vi "Process.vi"(8 "error in (no error)":errorcluster, 10 "pound in":refnum<class "Pound.lvclass">, 11 "qbus in":refnum<class "Qbus.lvclass">) -> (0 "error out":errorcluster)   [LabVIEW 2015, in "MainController.lvlib"]
doc: "Implements timer tasks that other processes register by sending Qbus messages to those processes."
uses:
  MainController.lvlib
  <vilib>/addons/Qbus/Qbus.lvclass
  <vilib>/NI/Software Watchdog/Pound/Pound.lvclass
  controls/ProcessState.ctl
  <vilib>/drjdpowell/SQLite Library/SQL Connection/Connection.lvclass
  <vilib>/NI/Software Watchdog/Watchdog/Watchdog.lvclass
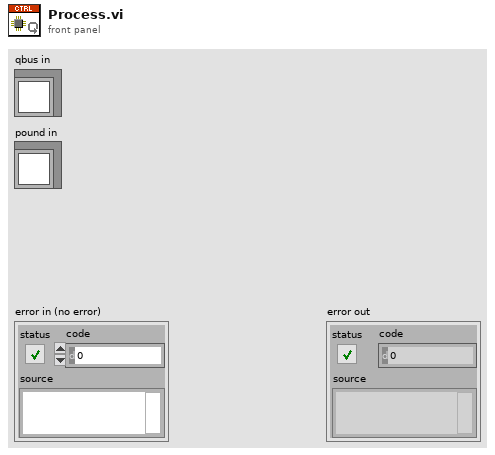
[diagram p1: front panel]
types:
  T1 = typedef "MainController.lvlib/ProcessState.ctl" = cluster{"SQLite Connection":refnum<class "Connection.lvclass">}
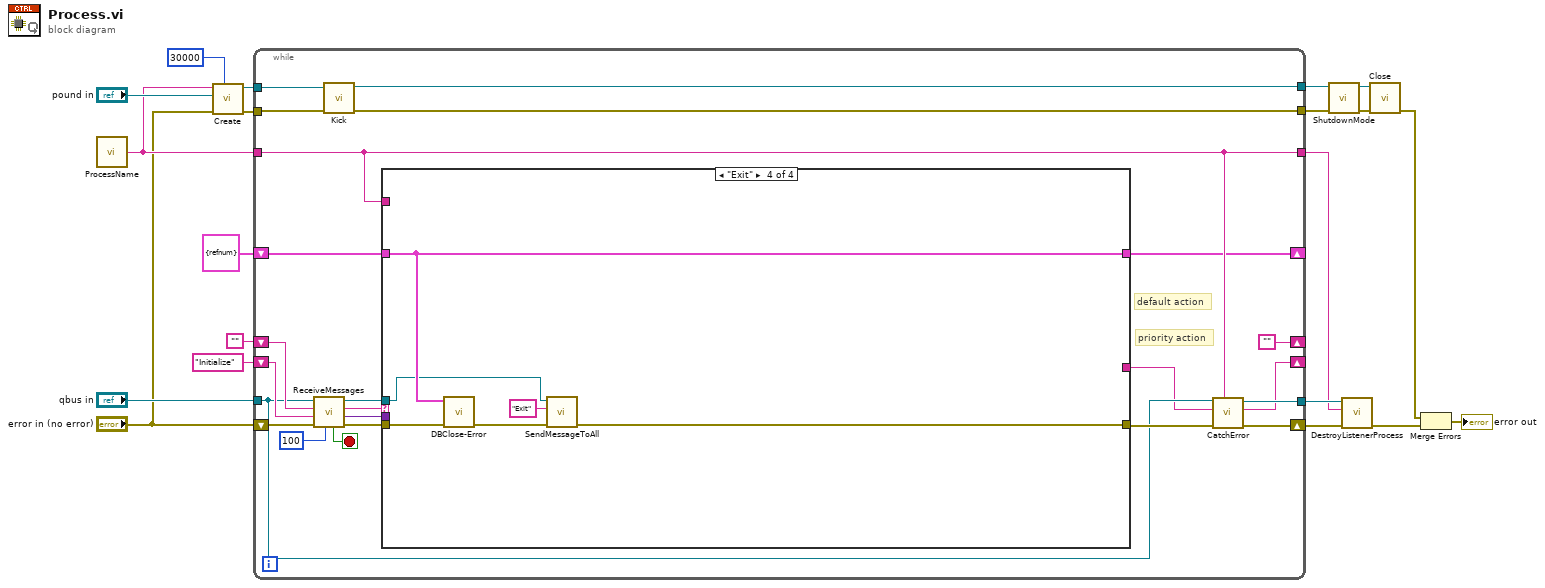
[diagram p0: block diagram]
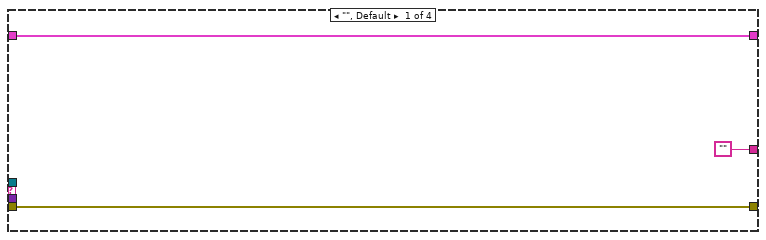
[diagram p2: hidden frame]
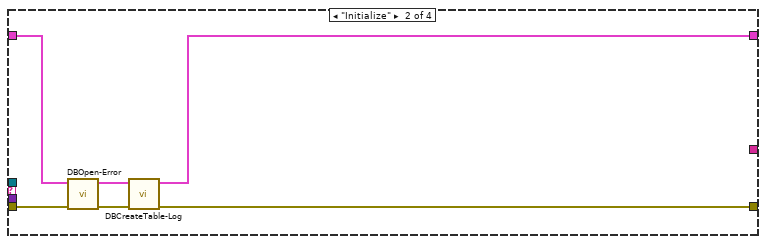
[diagram p3: hidden frame]
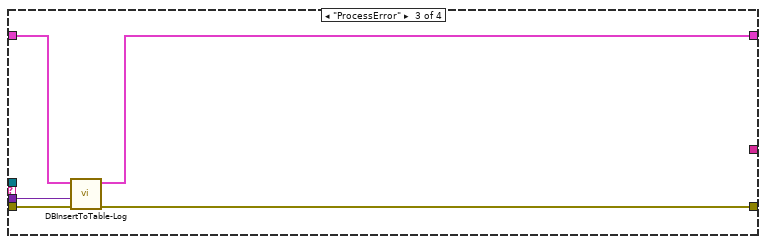
[diagram p4: hidden frame]
diagram:
  n1 = call "ProcessName.vi"() -> ("process name"=w11:string)  [unwired: 5 in]
  n2 = call <vilib>:"Create.vi"("Execution Timeout (ms)"=u32 30000, "error in (no error)"="error in (no error)", "Pound"="pound in", "Name"=w11) -> ("error out"=w13:errorcluster, "Watchdog"=w12:refnum<data-value>)  [unwired: 6 in]
  n3 = while {
    shift-right: [""] -> _
    shift-left: "" -> [w41]
    tunnel: "qbus in" -> [w25]
    tunnel: w11 -> [w32]
    tunnel: [w34] -> w18
    tunnel: [w32] -> w17
    shift-right: [w33] -> _
    shift-left: "Initialize" -> [w36]
    tunnel: w13 -> [w30]
    tunnel: w12 -> [w29]
    tunnel: [w28] -> w6
    tunnel: [w27] -> w7
    shift-right: [w35] -> w19
    shift-left: "error in (no error)" -> [w43]
    shift-right: [w22] -> _
    shift-left: T1 {"SQLite Connection"=refnum} ("ProcessState") -> [w23]
    stop <- w42 stop-if-true
    # "priority action"
    # "default action"
    n4 = call "ReceiveMessages.vi"("timeout(100)"=100, "error in (no error)"=w43, "priority action"=w36, "default action"=w41, "qbus in"=w25) -> ("error out"=w40:errorcluster, "message value"=w37:variant, "action"=w26:string, "qbus out"=w38:refnum<class "Qbus.lvclass">, "exit"=w42:bool)  [unwired: 2 in]
    n5 = call <vilib>:"Kick.vi"("error in (no error)"=w30, "Watchdog"=w29) -> ("error out"=w27:errorcluster, "Watchdog"=w28:refnum<data-value>)  [unwired: 8 in]
    n6 = case shown="\"Exit\"" w26 {
      tunnel: w40 -> [w46 w52 w57 w63]
      tunnel: w38 -> [_ _ _ w58]
      tunnel: [w46 w47 w53 w59] -> w31
      tunnel: w37 -> [_ _ w55 _]
      tunnel: w32 -> [_ _ _ _]
      tunnel: w23 -> [w45 w51 w56 w62]
      tunnel: [w45 w48 w54 w62] -> w22
      tunnel: ["" _ _ _] -> w21
      frame "", Default {
      }
      frame "Initialize" {
        n7 = call "DBOpen-Error.vi"("error in (no error)"=w52, "ProcessState in"=w51) -> ("error out"=w49:errorcluster, "ProcessState out"=w50:T1)  [unwired: 8 in]
        n8 = call "DBCreateTable-Log.vi"("error in (no error)"=w49, "ProcessState in"=w50) -> ("error out"=w47:errorcluster, "ProcessState out"=w48:T1)  [unwired: 8 in]
      }
      frame "ProcessError" {
        n9 = call "DBInsertToTable-Log.vi"("error in (no error)"=w57, "message value"=w55, "ProcessState in"=w56) -> ("error out"=w53:errorcluster, "ProcessState out"=w54:T1)  [unwired: 7 in]
      }
      frame "Exit" {
        n10 = call "DBClose-Error.vi"("error in (no error)"=w63, "ProcessState in"=w62) -> ("error out"=w60:errorcluster)  [unwired: 9 in]
        n11 = call <vilib>:"SendMessageToAll.vi"("error in (no error)"=w60, "message name"="Exit", "Qbus in"=w58) -> ("error in (no error)"=w59:errorcluster)  [unwired: 7 in, 1 out]
      }
    }
    n12 = call <vilib>:"CatchError.vi"("source"=w32, "error in (no error)"=w31, "next action in"=w21, "Qbus in"=w25) -> ("error out"=w35:errorcluster, "next action out"=w33:string, "Qbus out"=w34:refnum<class "Qbus.lvclass">)  [unwired: 5 in]
  }
  n13 = call <vilib>:"ShutdownMode.vi"("error in (no error)"=w7, "Watchdog"=w6) -> ("error out"=w8:errorcluster, "Watchdog"=w9:refnum<data-value>)  [unwired: 8 in]
  n14 = call <vilib>:"DestroyListenerProcess.vi"("error in (no error)"=w19, "process name"=w17, "Qbus in"=w18) -> ("error in (no error)"=w4:errorcluster)  [unwired: 7 in, 1 out]
  n15 = call <vilib>:"Close.vi"("error in (no error)"=w8, "Watchdog"=w9) -> ("error out"=w5:errorcluster)  [unwired: 9 in]
  n16 = Merge Errors(w5, w4) -> (→"error out":errorcluster)
